vi "Benchmark to String.vi"(7 "Divide/1k":bool, 11 "Timing Stats":T1) -> (3 "concatenated string":string)   [LabVIEW 2021, in "CIFCoreCommon.lvlib"]
uses:
  CIFCoreCommon.lvlib
  Typedef/Timing Stats Base.ctl
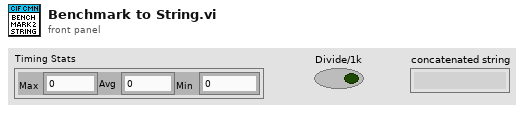
[diagram p1: front panel]
types:
  T1 = typedef "CIFCoreCommon.lvlib/Timing Stats Base.ctl" = cluster{"Max":i64, "Avg":dbl, "Min":i64}
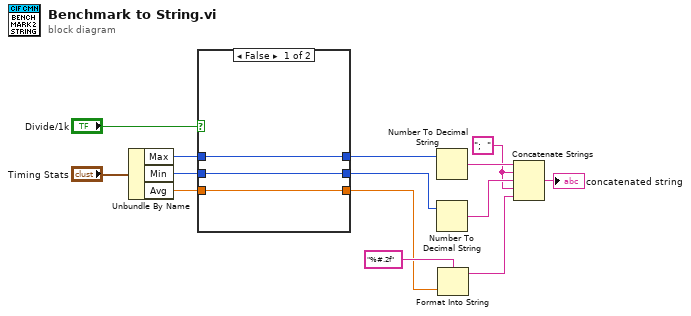
[diagram p0: block diagram]
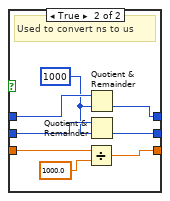
[diagram p2: hidden frame]
diagram:
  w9 = ";  "
  n1 = Unbundle By Name("Timing Stats") -> ("Max"=w7:i64, "Min"=w4:i64, "Avg"=w2:dbl)
  n2 = case shown="False" "Divide/1k" {
    tunnel: w7 -> [w17 w25]
    tunnel: [w17 w22] -> w6
    tunnel: [w16 w23] -> w5
    tunnel: w4 -> [w16 w24]
    tunnel: [w15 w19] -> w3
    tunnel: w2 -> [w15 w20]
    frame False {
    }
    frame True {
      w21 = i64 1000 ("y")
      # "Used to convert ns to us"
      n3 = Divide(x=w20, y=1000.0) -> (x/y=w19:dbl)
      n4 = Quotient & Remainder(x=w25, y=w21) -> (floor(x/y)=w22:i64)  [unwired: 1 out]
      n5 = Quotient & Remainder(x=w24, y=w21) -> (floor(x/y)=w23:i64)  [unwired: 1 out]
    }
  }
  n6 = Number To Decimal String(number=w6) -> (decimal integer string=w14:string)  [unwired: 1 in]
  n7 = Number To Decimal String(number=w5) -> (decimal integer string=w13:string)  [unwired: 1 in]
  n8 = Format Into String(format string="%#.2f", w3) -> (resulting string=w8:string)  [unwired: 2 in, 1 out]
  n9 = Concatenate Strings(w14, w9, w13, w9, w8) -> (→"concatenated string":string)
